vi "DIFF_DRIVE_ACT.vi"(8 "error in":errorcluster) -> (0 "error out":errorcluster)   [LabVIEW 2023]
uses:
  <vilib>/Rock Robotics/WPI/ThirdParty/Phoenix-LabVIEW/Motor Controller/Controls/CTRE_Phoenix_MotorControl_ControlMode.ctl
  <vilib>/Rock Robotics/WPI/ThirdParty/JAS_Junk/TrajLib/Trajectory_Library.lvlib
  <vilib>/Rock Robotics/WPI/ThirdParty/JAS_Junk/TrajLib/TypeDef/SIMPLE_MOTOR_FF.ctl
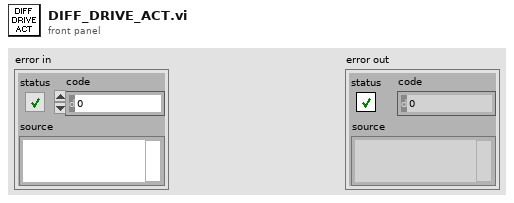
[diagram p1: front panel]
types:
  T1 = typedef "Trajectory_Library.lvlib/SIMPLE_MOTOR_FF.ctl" = cluster{"Ks":dbl, "Kv":dbl, "Ka":dbl, "KnInv":dbl}
  T2 = typedef "Trajectory_Library.lvlib/CHASSIS_SPEEDS.ctl" = cluster{"vX":dbl, "vY":dbl, "vOmega":dbl}
  T3 = typedef "Trajectory_Library.lvlib/DIFF_DRIVE_KINEMATICS.ctl" = cluster{"TrackWidth_Meters":dbl}
  T4 = enum16{"DemandType_Neutral", "DemandType_AuxPID", "DemandType_ArbitraryFeedForward"}
  T5 = typedef "CTRE_Phoenix_MotorControl_ControlMode.ctl" = u16
  T6 = typedef "WPI_MotorControlDeviceRef.ctl" = cluster{"DeviceStatus":errorcluster, "Type":T7, "PWM":cluster{"PWM Channel":T8, "DeadBand":T9}, "CAN":cluster{"Device Number":u8, "SetOutput VI Ref":variant, "GetOutput VI Ref":variant, "Enable VI Ref":variant, "Disable VI Ref":variant, "Data":variant}, "Invert":bool, "DIO PWM":cluster{"PWM \"Enable\" Channel":T8, "DIOChannel":T10, "PWM Rate":dbl}}
  T7 = typedef "WPI_MotorControlType.ctl" = enum16{"PWM", "CAN", "DIO PWM"}
  T8 = typedef "FPGA_DIOPWMChannel.ctl" = enum8{"PWM 0", "PWM 1", "PWM 2", "PWM 3", "PWM 4", "PWM 5", "PWM 6", "PWM 7", "PWM 8", "PWM 9", "PWM MXP 0", "PWM MXP 1", "PWM MXP 2", "PWM MXP 3", "PWM MXP 4", "PWM MXP 5", "PWM MXP 6", "PWM MXP 7", "PWM MXP 8", "PWM MXP 9", "Invalid"}
  T9 = typedef "WPI_PWMDeadband.ctl" = cluster{"Name":string, "maxPositivePwm":i32, "minPositivePwm":i32, "centerPwm":i32, "maxNegativePwm":i32, "minNegativePwm":i32, "angularRange":u16}
  T10 = typedef "FPGA_DIOChannel.ctl" = enum8{"DIO 0", "DIO 1", "DIO 2", "DIO 3", "DIO 4", "DIO 5", "DIO 6", "DIO 7", "DIO 8", "DIO 9", "DIO MXP 0", "DIO MXP 1", "DIO MXP 2", "DIO MXP 3", "DIO MXP 4", "DIO MXP 5", "DIO MXP 6", "DIO MXP 7", "DIO MXP 8", "DIO MXP 9", "DIO MXP 10", "DIO MXP 11", "DIO MXP 12", "DIO MXP 13", "DIO MXP 14", "DIO MXP 15", "SPI Port CS1", "SPI Port CS2", "SPI Port CS3", "SPI Port MISO", "SPI Port MOSI", "Invalid"}
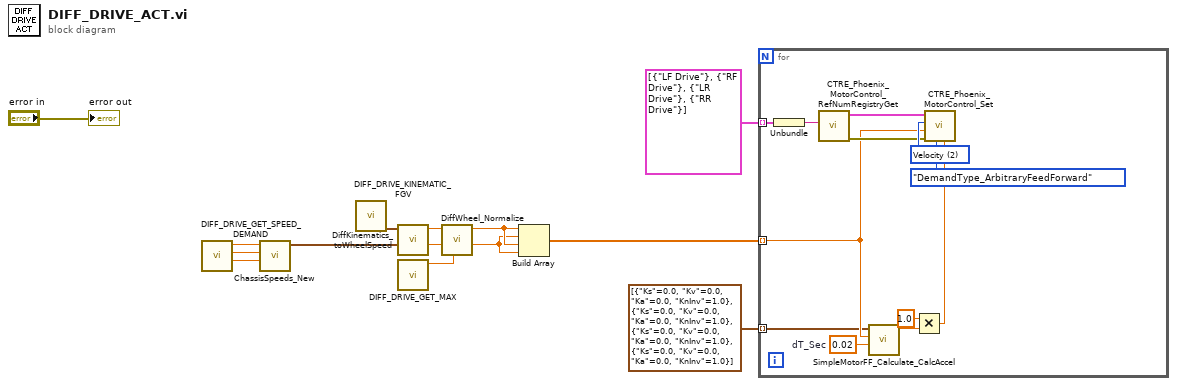
[diagram p0: block diagram]
diagram:
  n1 = call "DIFF_DRIVE_GET_SPEED_DEMAND.vi"() -> ("Drv Angular Vel Dmd"=w10:dbl, "Drv Y Vel Dmd"=w11:dbl, "Drv X Vel Dmd"=w12:dbl)  [unwired: 8 in, 1 out]
  n2 = call <vilib>:"ChassisSpeeds_New.vi"("vAngular"=w10, "vY"=w11, "vX"=w12) -> ("CHASSIS"=w9:T2)  [unwired: 8 in]
  n3 = call "DIFF_DRIVE_KINEMATIC_FGV.vi"() -> ("out DIFF_DRIVE_KINEMATICS"=w14:T3)  [unwired: 11 in]
  n4 = call <vilib>:"DiffKinematics_toWheelSpeed.vi"("CHASSIS Speed"=w9, "DIFF_DRIVE_KINEMATICS"=w14) -> ("RightVelocity"=w7:dbl, "LeftVelocity"=w8:dbl)  [unwired: 8 in]
  n5 = call "DIFF_DRIVE_GET_MAX.vi"() -> ("Max Wheel Vel (Meter/Sec)"=w6:dbl)  [unwired: 10 in, 1 out]
  n6 = call <vilib>:"DiffWheel_Normalize.vi"("Max Speed"=w6, "Right Wheel Demand"=w7, "Left Wheel Demand"=w8) -> ("Normalized Right Wheel Demand"=w4:dbl, "Normalized Left Wheel Demand"=w5:dbl)  [unwired: 7 in]
  n7 = Build Array(w5, w4, w5, w4) -> (w2:dbl[])
  n8 = for {
    tunnel: cluster{string}[] [{"LF Drive"}, {"RF Drive"}, {"LR Drive"}, {"RR Drive"}] -> [w22] mode=indexing
    tunnel: w2 -> [w20] mode=indexing
    tunnel: T1[] [{"Ks"=0.0, "Kv"=0.0, "Ka"=0.0, "KnInv"=1.0}, {"Ks"=0.0, "Kv"=0.0, "Ka"=0.0, "KnInv"=1.0}, {"Ks"=0.0, "Kv"=0.0, "Ka"=0.0, "KnInv"=1.0}, {"Ks"=0.0, "Kv"=0.0, "Ka"=0.0, "KnInv"=1.0}] -> [w19] mode=indexing
    w18 = 0.02  # dT_Sec
    w26 = T5 2 items=["PercentOutput"=0, "Position"=1, "Velocity"=2, "Current"=3, "Follower"=5, "MotionProfile"=6, "MotionMagic"=7, "MotionProfileArc"=10, "Disabled"=15] ("Control Mode")
    n9 = Unbundle(w22) -> (w21:string)
    n10 = call <vilib>:"CTRE_Phoenix_MotorControl_RefNumRegistryGet.vi"("refnum name"=w21) -> ("error out"=w25:errorcluster, "PhoenixMotorControlDevRef"=w24:T6)  [unwired: 9 in]
    n11 = call <vilib>:"SimpleMotorFF_Calculate_CalcAccel.vi"("dT_Sec"=w18, "VelSp"=w20, "SIMPLE_MOTOR_FF"=w19) -> ("FeedForward"=w17:dbl)  [unwired: 8 in]
    n12 = Multiply(x=1.0, y=w17) -> (x*y=w16:dbl)
    n13 = call <vilib>:"CTRE_Phoenix_MotorControl_Set.vi"("Demand1"=w16, "DemandType"=T4."DemandType_ArbitraryFeedForward", "error in (no error)"=w25, "Output"=w20, "Control Mode"=w26, "PhoenixMotorControlDevRef"=w24) -> ()  [unwired: 4 in, 2 out]
  }
  "error out" <- "error in"
